vi "MPUInit.vi"(6 "Timeout (10 s)":u8=10, 8 "ErrorIn(no error)":errorcluster, 11 "FPGA VI引用输入":refnum<k20>) -> (0 "ErrorOut":errorcluster, 3 "FPGA VI引用输出":refnum<k20>)   [LabVIEW 2015]
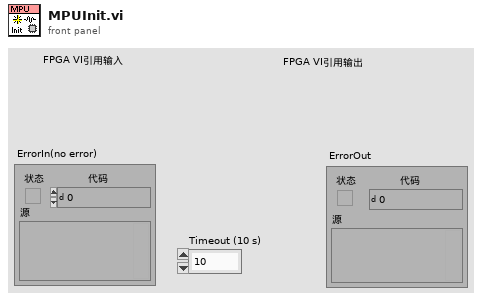
[diagram p1: front panel]
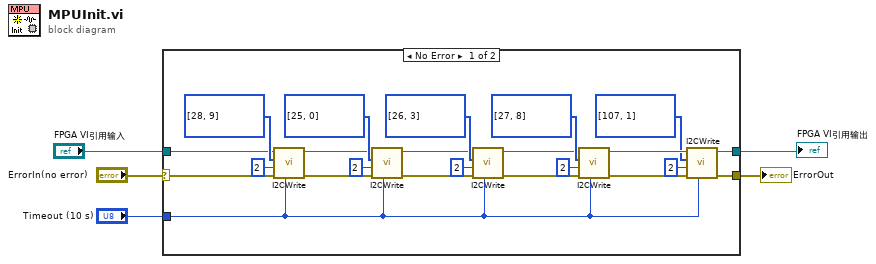
[diagram p0: block diagram]
diagram:
  n1 = case shown="No Error" "ErrorIn(no error)" {
    selector: "ErrorIn(no error)" -> [w9 w29]
    tunnel: "FPGA VI引用输入" -> [w10 w30]
    tunnel: [w8 w30] -> w1
    tunnel: [w7 w29] -> w4
    tunnel: "Timeout (10 s)" -> [w6 _]
    frame No Error {
      n2 = call "I2CWrite.vi"("Timeout (10 s)"=w6, "error in (no error)"=w9, "Number of Bytes to Write"=u8 2, "Data"=u8[] [28, 9], "FPGA VI引用输入"=w10) -> ("error out"=w24:errorcluster, "FPGA VI引用输出"=w25:refnum<k20>)  [unwired: 5 in]
      n3 = call "I2CWrite.vi"("Timeout (10 s)"=w6, "error in (no error)"=w24, "Number of Bytes to Write"=u8 2, "Data"=u8[] [25, 0], "FPGA VI引用输入"=w25) -> ("error out"=w21:errorcluster, "FPGA VI引用输出"=w20:refnum<k20>)  [unwired: 5 in]
      n4 = call "I2CWrite.vi"("Timeout (10 s)"=w6, "error in (no error)"=w21, "Number of Bytes to Write"=u8 2, "Data"=u8[] [26, 3], "FPGA VI引用输入"=w20) -> ("error out"=w16:errorcluster, "FPGA VI引用输出"=w17:refnum<k20>)  [unwired: 5 in]
      n5 = call "I2CWrite.vi"("Timeout (10 s)"=w6, "error in (no error)"=w16, "Number of Bytes to Write"=u8 2, "Data"=u8[] [27, 8], "FPGA VI引用输入"=w17) -> ("error out"=w13:errorcluster, "FPGA VI引用输出"=w14:refnum<k20>)  [unwired: 5 in]
      n6 = call "I2CWrite.vi"("Timeout (10 s)"=w6, "error in (no error)"=w13, "Number of Bytes to Write"=u8 2, "Data"=u8[] [107, 1], "FPGA VI引用输入"=w14) -> ("error out"=w7:errorcluster, "FPGA VI引用输出"=w8:refnum<k20>)  [unwired: 5 in]
    }
    frame Error {
    }
  }
  "ErrorOut" <- w4
  "FPGA VI引用输出" <- w1
